vi "Autonomous Independent.vi"   [LabVIEW 2019]
doc: "This VI is called when autonomous begins, and will automatically be terminated when autonomous ends. You can carry out timed or sensor driven robot movement independently without needing to return to the caller."
uses:
  <vilib>/Rock Robotics/WPI/Utilities/WPI_GetSetVariantRefNum.vi
  <vilib>/Rock Robotics/Network Tables/NT Read String.vi
  <vilib>/Rock Robotics/Network Tables/NT Write Numeric Array.vi
  Robot Global Data.vi
panel:
  # "Be sure to right-click and choose Data Operations>>Make Current Value default if you want to save the array values with the VI"
types:
  T1 = typedef "WPI_JoystickDevRef.ctl" = cluster{"Device":T2}
  T2 = typedef "WPI_JoystickDeviceEnum.ctl" = enum16{"USB 0", "USB 1", "USB 2", "USB 3", "USB 4", "USB 5"}
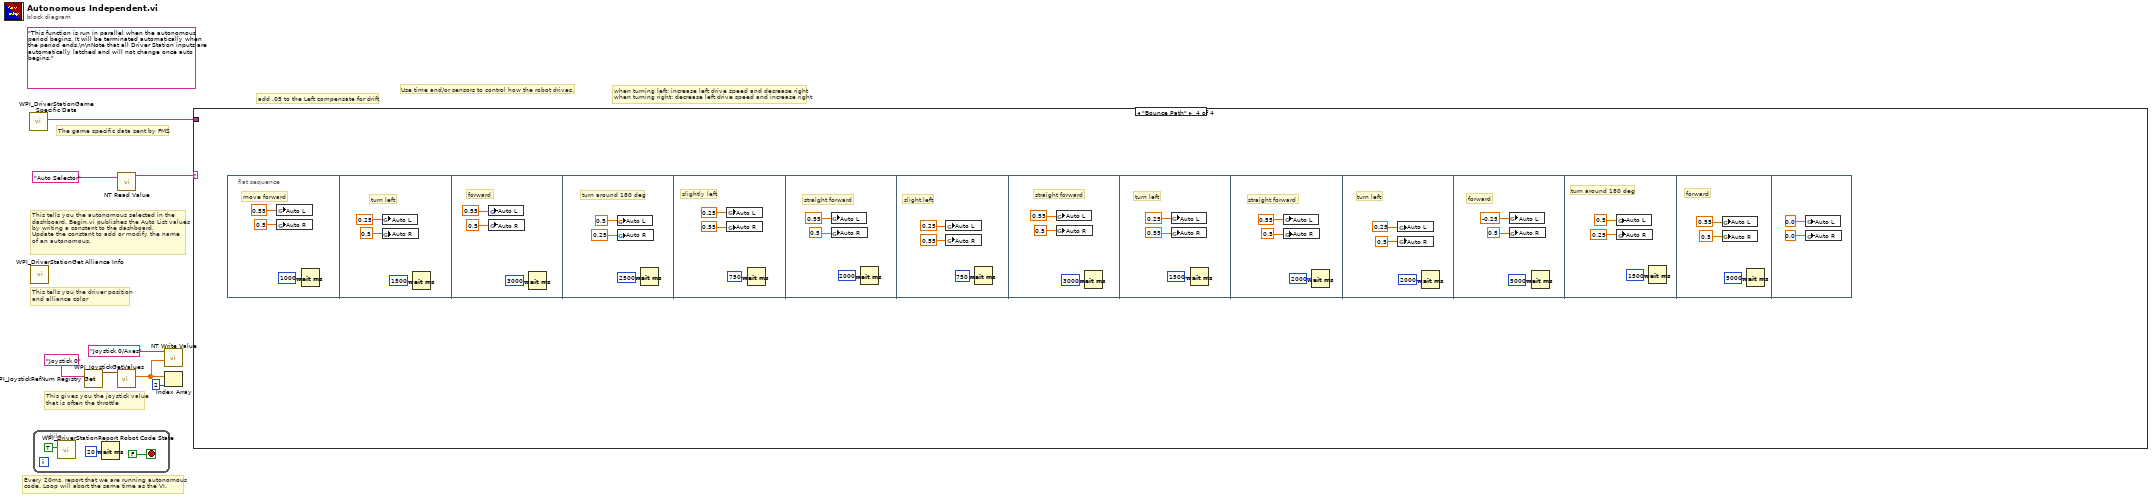
[diagram p0: block diagram]
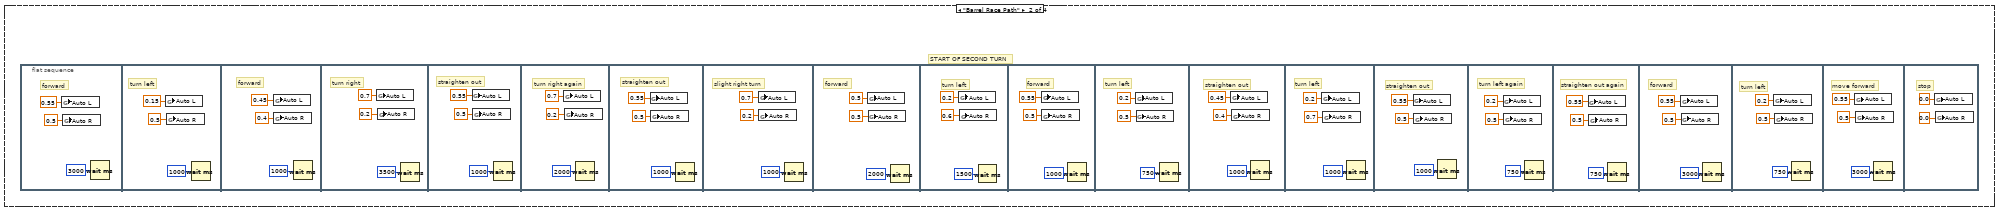
[diagram p3: hidden frame]
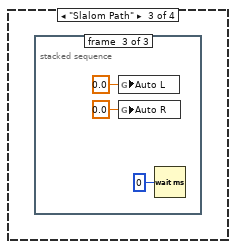
[diagram p4: hidden frame]
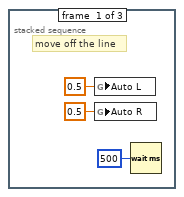
[diagram p5: hidden frame]
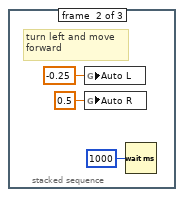
[diagram p6: hidden frame]
diagram:
  (unwired) "This function is run in parallel when the autonomous period begins. It will be terminated automatically when the period ends.\n\nNote that all Driver Station inputs are automatically latched and will not change once auto begins."
  # "add .05 to the Left compensate for drift"
  # "when turning left: increase left drive speed and decrease right\nwhen turning right: decrease left drive speed and increase right"
  # "The game specific data sent by FMS"
  # "This tells you the autonomous selected in the \ndashboard. Begin.vi publishes the Auto List values\nby writing a constant to the dashboard.\nUpdate the constant to add or modify the name\nof an autonomous."
  # "Every 20ms, report that we are running autonomous\ncode. Loop will abort the same time as the VI."
  # "This gives you the joystick value\nthat is often the throttle"
  # "Use time and/or sensors to control how the robot drives."
  # "This tells you the driver position\nand alliance color"
  n1 = call <vilib>:"WPI_DriverStationGame Specific Data.vi"() -> ("Game Specific Data"=w1:string)  [unwired: 11 in]
  n2 = call <vilib>:"WPI_DriverStationGet Alliance Info.vi"() -> ()  [unwired: 12 out]
  n3 = while {
    stop <- FALSE stop-if-true
    n4 = call <vilib>:"WPI_DriverStationReport Robot Code State.vi"("Autonomous"=TRUE) -> ()  [unwired: 10 in, 1 out]
    n5 = Wait (ms)(milliseconds to wait=u32 20) -> ()  [unwired: 1 out]
  }
  n6 = call <vilib>:"WPI_JoystickRefNum Registry Get.vi"("refnum name"="Joystick 0") -> ("JoystickDevRef"=w7:T1)  [unwired: 1 in, 9 out]
  n7 = call <vilib>:"WPI_JoystickGetValues.vi"("JoystickDevRef"=w7) -> ("Axes"=w3:dbl[])  [unwired: 6 in, 4 out]
  n8 = call-poly <vilib>:"NT Read Value.vi"("Name"="Auto Selector") -> ("String"=w4:string)  [unwired: 9 in, 1 out]
  n9 = call-poly <vilib>:"NT Write Value.vi"("Numeric Array"=w3, "Name"="Joystick 0/Axes") -> ()  [unwired: 9 in, 1 out]
  n10 = Index Array(array=w3, index=2) -> ()  [unwired: 1 out]
  n11 = case shown="\"Bounce Path\"" w4 {
    tunnel: w1 -> [_ _ _ _]
    frame Default {
      # "You can put your main auto here, or you can right-click on the case and make any\nother frame be the default case."
      # "This is the frame that will execute if no selection is made, or if it is not recognized"
    }
    frame "Barrel Race Path" {
      # "START OF SECOND TURN"
      n12 = flat-sequence {
        frame #0 {
          # "forward"
          n13 = global write "Robot Global Data.vi" "Auto L"(0.55 ("Auto X")) -> ()
          n14 = global write "Robot Global Data.vi" "Auto R"(0.5 ("Auto Y")) -> ()
          n15 = Wait (ms)(milliseconds to wait=u32 3000) -> ()  [unwired: 1 out]
        }
        frame #1 {
          # "turn left"
          n16 = global write "Robot Global Data.vi" "Auto L"(0.15 ("Auto X")) -> ()
          n17 = global write "Robot Global Data.vi" "Auto R"(0.5 ("Auto Y")) -> ()
          n18 = Wait (ms)(milliseconds to wait=u32 1000) -> ()  [unwired: 1 out]
        }
        frame #2 {
          # "forward"
          n19 = global write "Robot Global Data.vi" "Auto L"(0.45 ("Auto X")) -> ()
          n20 = global write "Robot Global Data.vi" "Auto R"(0.4 ("Auto Y")) -> ()
          n21 = Wait (ms)(milliseconds to wait=u32 1000) -> ()  [unwired: 1 out]
        }
        frame #3 {
          # "turn right"
          n22 = global write "Robot Global Data.vi" "Auto L"(0.7 ("Auto X")) -> ()
          n23 = global write "Robot Global Data.vi" "Auto R"(0.2 ("Auto Y")) -> ()
          n24 = Wait (ms)(milliseconds to wait=u32 3500) -> ()  [unwired: 1 out]
        }
        frame #4 {
          # "straighten out"
          n25 = global write "Robot Global Data.vi" "Auto L"(0.55 ("Auto X")) -> ()
          n26 = global write "Robot Global Data.vi" "Auto R"(0.5 ("Auto Y")) -> ()
          n27 = Wait (ms)(milliseconds to wait=u32 1000) -> ()  [unwired: 1 out]
        }
        frame #5 {
          # "turn right again"
          n28 = global write "Robot Global Data.vi" "Auto L"(0.7 ("Auto X")) -> ()
          n29 = global write "Robot Global Data.vi" "Auto R"(0.2 ("Auto Y")) -> ()
          n30 = Wait (ms)(milliseconds to wait=u32 2000) -> ()  [unwired: 1 out]
        }
        frame #6 {
          # "straighten out"
          n31 = global write "Robot Global Data.vi" "Auto L"(0.55 ("Auto X")) -> ()
          n32 = global write "Robot Global Data.vi" "Auto R"(0.5 ("Auto Y")) -> ()
          n33 = Wait (ms)(milliseconds to wait=u32 1000) -> ()  [unwired: 1 out]
        }
        frame #7 {
          # "slight right turn"
          n34 = global write "Robot Global Data.vi" "Auto L"(0.7 ("Auto X")) -> ()
          n35 = global write "Robot Global Data.vi" "Auto R"(0.2 ("Auto Y")) -> ()
          n36 = Wait (ms)(milliseconds to wait=u32 1000) -> ()  [unwired: 1 out]
        }
        frame #8 {
          # "forward"
          n37 = global write "Robot Global Data.vi" "Auto L"(0.5 ("Auto X")) -> ()
          n38 = global write "Robot Global Data.vi" "Auto R"(0.5 ("Auto Y")) -> ()
          n39 = Wait (ms)(milliseconds to wait=u32 2000) -> ()  [unwired: 1 out]
        }
        frame #9 {
          # "turn left"
          n40 = global write "Robot Global Data.vi" "Auto L"(0.2 ("Auto X")) -> ()
          n41 = global write "Robot Global Data.vi" "Auto R"(0.6 ("Auto Y")) -> ()
          n42 = Wait (ms)(milliseconds to wait=u32 1500) -> ()  [unwired: 1 out]
        }
        frame #10 {
          # "forward"
          n43 = global write "Robot Global Data.vi" "Auto L"(0.55 ("Auto X")) -> ()
          n44 = global write "Robot Global Data.vi" "Auto R"(0.5 ("Auto Y")) -> ()
          n45 = Wait (ms)(milliseconds to wait=u32 1000) -> ()  [unwired: 1 out]
        }
        frame #11 {
          # "turn left"
          n46 = global write "Robot Global Data.vi" "Auto L"(0.2 ("Auto X")) -> ()
          n47 = global write "Robot Global Data.vi" "Auto R"(0.5 ("Auto Y")) -> ()
          n48 = Wait (ms)(milliseconds to wait=u32 750) -> ()  [unwired: 1 out]
        }
        frame #12 {
          # "straighten out"
          n49 = global write "Robot Global Data.vi" "Auto L"(0.45 ("Auto X")) -> ()
          n50 = global write "Robot Global Data.vi" "Auto R"(0.4 ("Auto Y")) -> ()
          n51 = Wait (ms)(milliseconds to wait=u32 1000) -> ()  [unwired: 1 out]
        }
        frame #13 {
          # "turn left"
          n52 = global write "Robot Global Data.vi" "Auto L"(0.2 ("Auto X")) -> ()
          n53 = global write "Robot Global Data.vi" "Auto R"(0.7 ("Auto Y")) -> ()
          n54 = Wait (ms)(milliseconds to wait=u32 1000) -> ()  [unwired: 1 out]
        }
        frame #14 {
          # "straighten out"
          n55 = global write "Robot Global Data.vi" "Auto L"(0.55 ("Auto X")) -> ()
          n56 = global write "Robot Global Data.vi" "Auto R"(0.5 ("Auto Y")) -> ()
          n57 = Wait (ms)(milliseconds to wait=u32 1000) -> ()  [unwired: 1 out]
        }
        frame #15 {
          # "turn left again"
          n58 = global write "Robot Global Data.vi" "Auto L"(0.2 ("Auto X")) -> ()
          n59 = global write "Robot Global Data.vi" "Auto R"(0.5 ("Auto Y")) -> ()
          n60 = Wait (ms)(milliseconds to wait=u32 750) -> ()  [unwired: 1 out]
        }
        frame #16 {
          # "straighten out again"
          n61 = global write "Robot Global Data.vi" "Auto L"(0.55 ("Auto X")) -> ()
          n62 = global write "Robot Global Data.vi" "Auto R"(0.5 ("Auto Y")) -> ()
          n63 = Wait (ms)(milliseconds to wait=u32 750) -> ()  [unwired: 1 out]
        }
        frame #17 {
          # "forward"
          n64 = global write "Robot Global Data.vi" "Auto L"(0.55 ("Auto X")) -> ()
          n65 = global write "Robot Global Data.vi" "Auto R"(0.5 ("Auto Y")) -> ()
          n66 = Wait (ms)(milliseconds to wait=u32 3000) -> ()  [unwired: 1 out]
        }
        frame #18 {
          # "turn left"
          n67 = global write "Robot Global Data.vi" "Auto L"(0.2 ("Auto X")) -> ()
          n68 = global write "Robot Global Data.vi" "Auto R"(0.5 ("Auto Y")) -> ()
          n69 = Wait (ms)(milliseconds to wait=u32 750) -> ()  [unwired: 1 out]
        }
        frame #19 {
          # "move forward"
          n70 = global write "Robot Global Data.vi" "Auto L"(0.55 ("Auto X")) -> ()
          n71 = global write "Robot Global Data.vi" "Auto R"(0.5 ("Auto Y")) -> ()
          n72 = Wait (ms)(milliseconds to wait=u32 3000) -> ()  [unwired: 1 out]
        }
        frame #20 {
          # "stop"
          n73 = global write "Robot Global Data.vi" "Auto L"(0.0 ("Auto X")) -> ()
          n74 = global write "Robot Global Data.vi" "Auto R"(0.0 ("Auto Y")) -> ()
        }
      }
    }
    frame "Slalom Path" {
      n75 = stacked-sequence {
        frame #0 {
          # "move off the line"
          n76 = global write "Robot Global Data.vi" "Auto L"(0.5 ("Auto X")) -> ()
          n77 = global write "Robot Global Data.vi" "Auto R"(0.5 ("Auto Y")) -> ()
          n78 = Wait (ms)(milliseconds to wait=u32 500) -> ()  [unwired: 1 out]
        }
        frame #1 {
          # "turn left and move \nforward"
          n79 = global write "Robot Global Data.vi" "Auto L"(-0.25 ("Auto X")) -> ()
          n80 = global write "Robot Global Data.vi" "Auto R"(0.5 ("Auto Y")) -> ()
          n81 = Wait (ms)(milliseconds to wait=u32 1000) -> ()  [unwired: 1 out]
        }
        frame #2 {
          n82 = global write "Robot Global Data.vi" "Auto L"(0.0 ("Auto X")) -> ()
          n83 = global write "Robot Global Data.vi" "Auto R"(0.0 ("Auto Y")) -> ()
          n84 = Wait (ms)(milliseconds to wait=u32 0) -> ()  [unwired: 1 out]
        }
      }
    }
    frame "Bounce Path" {
      n85 = flat-sequence {
        frame #0 {
          # "move forward"
          n86 = global write "Robot Global Data.vi" "Auto L"(0.55 ("Joystick X")) -> ()
          n87 = global write "Robot Global Data.vi" "Auto R"(0.5 ("Joystick Y")) -> ()
          n88 = Wait (ms)(milliseconds to wait=u32 1000) -> ()  [unwired: 1 out]
        }
        frame #1 {
          # "turn left"
          n89 = global write "Robot Global Data.vi" "Auto L"(0.25 ("Joystick X")) -> ()
          n90 = global write "Robot Global Data.vi" "Auto R"(0.5 ("Joystick Y")) -> ()
          n91 = Wait (ms)(milliseconds to wait=u32 1500) -> ()  [unwired: 1 out]
        }
        frame #2 {
          # "forward"
          n92 = global write "Robot Global Data.vi" "Auto L"(0.55 ("Joystick X")) -> ()
          n93 = global write "Robot Global Data.vi" "Auto R"(0.5 ("Joystick Y")) -> ()
          n94 = Wait (ms)(milliseconds to wait=u32 3000) -> ()  [unwired: 1 out]
        }
        frame #3 {
          # "turn around 180 deg"
          n95 = global write "Robot Global Data.vi" "Auto L"(0.5 ("Joystick X")) -> ()
          n96 = global write "Robot Global Data.vi" "Auto R"(0.25 ("Joystick Y")) -> ()
          n97 = Wait (ms)(milliseconds to wait=u32 2500) -> ()  [unwired: 1 out]
        }
        frame #4 {
          # "slightly left"
          n98 = global write "Robot Global Data.vi" "Auto L"(0.25 ("Joystick X")) -> ()
          n99 = global write "Robot Global Data.vi" "Auto R"(0.55 ("Joystick Y")) -> ()
          n100 = Wait (ms)(milliseconds to wait=u32 750) -> ()  [unwired: 1 out]
        }
        frame #5 {
          # "straight forward"
          n101 = global write "Robot Global Data.vi" "Auto L"(0.55 ("Joystick X")) -> ()
          n102 = global write "Robot Global Data.vi" "Auto R"(0.5 ("Joystick Y")) -> ()
          n103 = Wait (ms)(milliseconds to wait=u32 2000) -> ()  [unwired: 1 out]
        }
        frame #6 {
          # "slight left"
          n104 = global write "Robot Global Data.vi" "Auto L"(0.25 ("Joystick X")) -> ()
          n105 = global write "Robot Global Data.vi" "Auto R"(0.55 ("Joystick Y")) -> ()
          n106 = Wait (ms)(milliseconds to wait=u32 750) -> ()  [unwired: 1 out]
        }
        frame #7 {
          # "straight forward"
          n107 = global write "Robot Global Data.vi" "Auto L"(0.55 ("Joystick X")) -> ()
          n108 = global write "Robot Global Data.vi" "Auto R"(0.5 ("Joystick Y")) -> ()
          n109 = Wait (ms)(milliseconds to wait=u32 3000) -> ()  [unwired: 1 out]
        }
        frame #8 {
          # "turn left"
          n110 = global write "Robot Global Data.vi" "Auto L"(0.25 ("Joystick X")) -> ()
          n111 = global write "Robot Global Data.vi" "Auto R"(0.55 ("Joystick Y")) -> ()
          n112 = Wait (ms)(milliseconds to wait=u32 1500) -> ()  [unwired: 1 out]
        }
        frame #9 {
          # "straight forward"
          n113 = global write "Robot Global Data.vi" "Auto L"(0.55 ("Joystick X")) -> ()
          n114 = global write "Robot Global Data.vi" "Auto R"(0.5 ("Joystick Y")) -> ()
          n115 = Wait (ms)(milliseconds to wait=u32 2000) -> ()  [unwired: 1 out]
        }
        frame #10 {
          # "turn left"
          n116 = global write "Robot Global Data.vi" "Auto L"(0.25 ("Joystick X")) -> ()
          n117 = global write "Robot Global Data.vi" "Auto R"(0.5 ("Joystick Y")) -> ()
          n118 = Wait (ms)(milliseconds to wait=u32 2000) -> ()  [unwired: 1 out]
        }
        frame #11 {
          # "forward"
          n119 = global write "Robot Global Data.vi" "Auto L"(-0.25 ("Joystick X")) -> ()
          n120 = global write "Robot Global Data.vi" "Auto R"(0.5 ("Joystick Y")) -> ()
          n121 = Wait (ms)(milliseconds to wait=u32 5000) -> ()  [unwired: 1 out]
        }
        frame #12 {
          # "turn around 180 deg"
          n122 = global write "Robot Global Data.vi" "Auto L"(0.5 ("Joystick X")) -> ()
          n123 = global write "Robot Global Data.vi" "Auto R"(0.25 ("Joystick Y")) -> ()
          n124 = Wait (ms)(milliseconds to wait=u32 1500) -> ()  [unwired: 1 out]
        }
        frame #13 {
          # "forward"
          n125 = global write "Robot Global Data.vi" "Auto L"(0.55 ("Joystick X")) -> ()
          n126 = global write "Robot Global Data.vi" "Auto R"(0.5 ("Joystick Y")) -> ()
          n127 = Wait (ms)(milliseconds to wait=u32 5000) -> ()  [unwired: 1 out]
        }
        frame #14 {
          n128 = global write "Robot Global Data.vi" "Auto L"(0.0 ("Joystick X")) -> ()
          n129 = global write "Robot Global Data.vi" "Auto R"(0.0 ("Joystick Y")) -> ()
        }
      }
    }
  }
